vi "InAs TED Characterise - PicoAmmeter.vi"() -> ()   [LabVIEW 2024]
uses:
  <vilib>/Analysis/1siggen.llb/Ramp Pattern by Delta.vi
  <instrlib>/Keithley 648X Series/Keithley 648X Series.lvlib
  <vilib>/Analysis/NI_AALBase.lvlib
panel:
  out "InAs Detector Response":cluster{"Ramp Pattern":dbl[], dbl[]}(graph)
  in  "Tdelta":dbl=1.0 format="%#_13g"
  in  "TFinish":dbl
  in  "TStart":dbl=-65.0
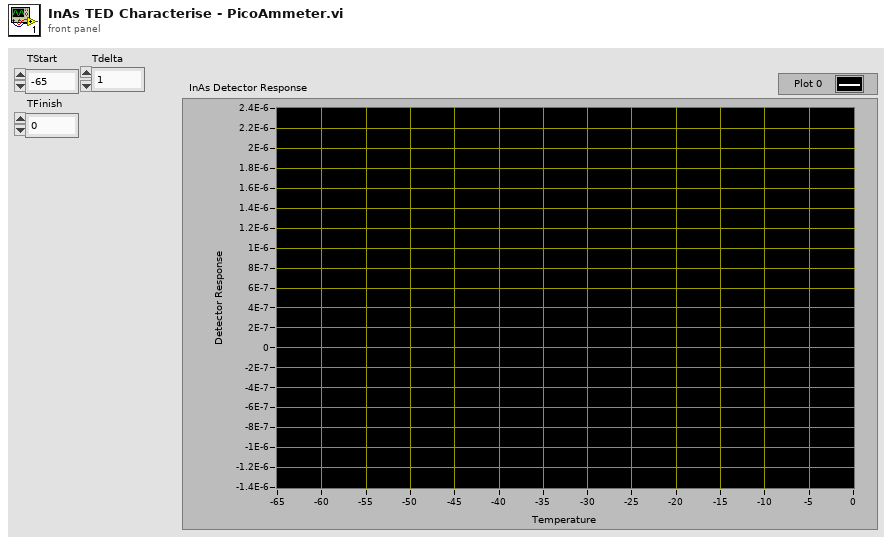
[diagram p1: front panel]
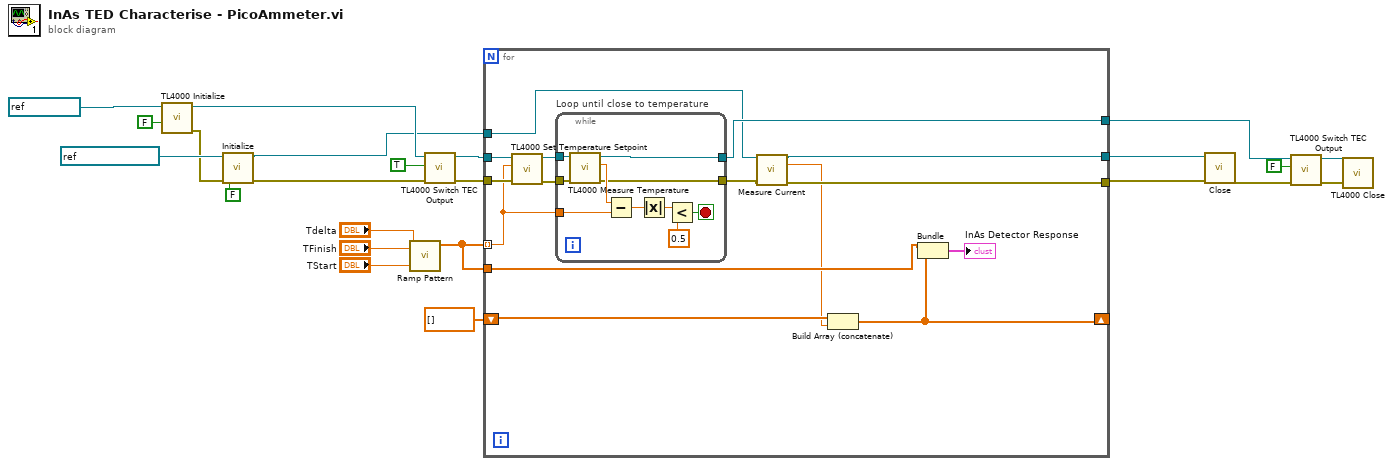
[diagram p0: block diagram]
diagram:
  n1 = call <instrlib>:"TL4000 Initialize.vi"("Reset Device (Reset Device)"=FALSE, "resource name"=refnum<visa-resource-name> "TED4015") -> ("error out"=w20:errorcluster, "instrument handle out"=w23:refnum<visa-resource-name>)  [unwired: 8 in]
  n2 = call <instrlib>:"Initialize.vi"("error in (no error)"=w20, "ID Query (True)"=FALSE ("Reset (True)"), "VISA resource name"=refnum<visa-resource-name> "Picoammeter") -> ("error out"=w1:errorcluster, "VISA resource name out"=w2:refnum<visa-resource-name>)  [unwired: 7 in]
  n3 = call-poly <vilib>:"Ramp Pattern.vi"("start"="TStart", "end"="TFinish", "delta"="Tdelta") -> ("Ramp Pattern"=w5:dbl[])  [unwired: 6 in, 2 out]
  n4 = call <instrlib>:"TL4000 Switch TEC Output.vi"("error in (no error)"=w1, "TEC Output (Off)"=TRUE, "instrument handle"=w23) -> ("error out"=w15:errorcluster, "instrument handle out"=w14:refnum<visa-resource-name>)  [unwired: 7 in]
  n5 = for {
    tunnel: w14 -> [w38]
    tunnel: w15 -> [w37]
    tunnel: w5 -> [w36] mode=indexing
    tunnel: w2 -> [w27]
    tunnel: [w25] -> w12
    tunnel: [w28] -> w13
    tunnel: [w33] -> w9
    shift-right: [w29] -> _
    shift-left: dbl[] [] -> [w32]
    tunnel: w5 -> [w30]
    n6 = call <instrlib>:"TL4000 Set Temperature Setpoint.vi"("error in (no error)"=w37, "Temperature Setpoint (25.0)"=w36, "instrument handle"=w38) -> ("error out"=w34:errorcluster, "instrument handle out"=w35:refnum<visa-resource-name>)  [unwired: 7 in]
    n7 = while "Loop until close to temperature" {
      tunnel: w34 -> [w42]
      tunnel: w35 -> [w43]
      tunnel: [w41] -> w33
      tunnel: [w39] -> w26
      tunnel: w36 -> [w48]
      stop <- w44 stop-if-true
      n8 = call <instrlib>:"TL4000 Measure Temperature.vi"("error in (no error)"=w42, "instrument handle"=w43) -> ("error out"=w39:errorcluster, "Temperature"=w40:dbl, "instrument handle out"=w41:refnum<visa-resource-name>)  [unwired: 7 in]
      n9 = Subtract(x=w40, y=w48) -> (x-y=w47:dbl)
      n10 = Absolute Value(x=w47) -> (abs(x)=w46:dbl)
      n11 = Less?(x=w46, y=0.5) -> (x < y?=w44:bool)
    }
    n12 = call <instrlib>:"Measure Current.vi"("VISA resource name"=w27, "error in (no error)"=w26) -> ("VISA resource name out"=w28:refnum<visa-resource-name>, "Measurement"=w24:dbl, "error out"=w25:errorcluster)  [unwired: 11 in]
    n13 = Build Array (concatenate)(w32, w24) -> (w29:dbl[])
    n14 = Bundle("Ramp Pattern"=w30, w29) -> (→"InAs Detector Response":cluster{"Ramp Pattern":dbl[], dbl[]})  [unwired: 1 in]
  }
  n15 = call <instrlib>:"Close.vi"("error in (no error)"=w12, "VISA resource name"=w13) -> ("error out"=w10:errorcluster)  [unwired: 9 in]
  n16 = call <instrlib>:"TL4000 Switch TEC Output.vi"("error in (no error)"=w10, "TEC Output (Off)"=FALSE, "instrument handle"=w9) -> ("error out"=w11:errorcluster, "instrument handle out"=w7:refnum<visa-resource-name>)  [unwired: 7 in]
  n17 = call <instrlib>:"TL4000 Close.vi"("error in (no error)"=w11, "instrument handle"=w7) -> ()  [unwired: 9 in, 1 out]
